vi "ngi request data.vi"(3 "stop":u32, 5 "start":u32, 6 "MAC source":string="\u0000\u0017\r\u0000\u0000`#Ò", 7 "Channels":u8, 8 "error in (no error)":errorcluster, 10 "this instance?":bool=TRUE, 11 "ID":u16) -> (0 "error out":errorcluster)   [LabVIEW 2017]
panel:
  out "concatenated string":string
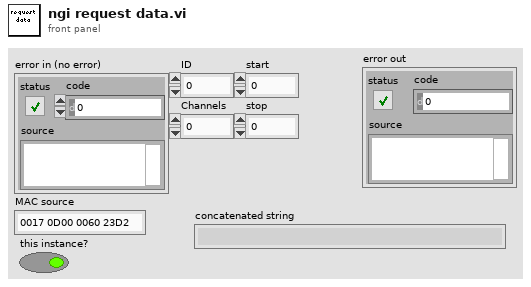
[diagram p1: front panel]
types:
  T1 = cluster{"ID":u16, "Channels":u8, "start":u32, "stop":u32}
  T2 = enum16{"big-endian, network order", "native, host order", "little-endian"}
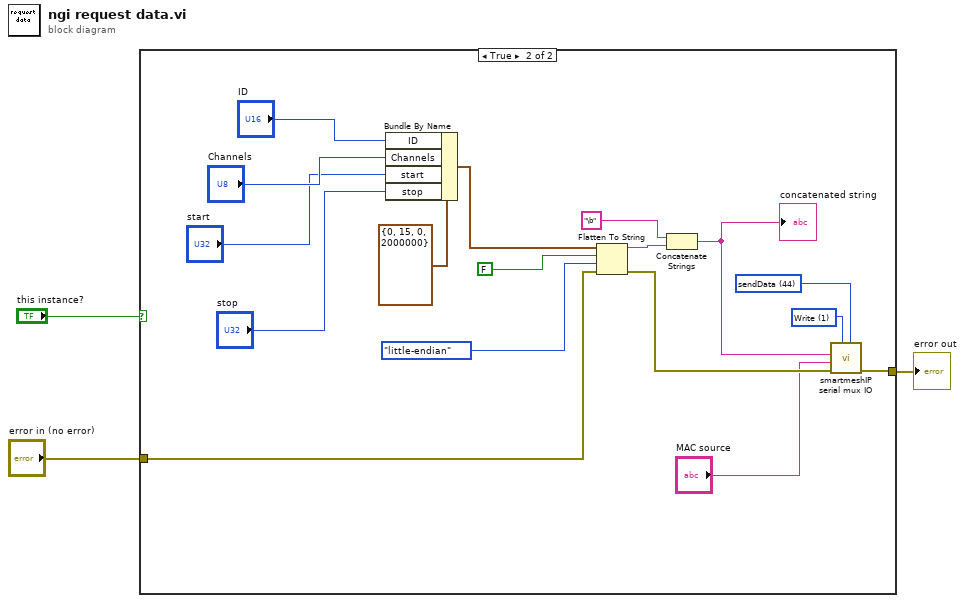
[diagram p0: block diagram]
diagram:
  n1 = case shown="True" "this instance?" {
    tunnel: [w4 w11] -> w3
    tunnel: "error in (no error)" -> [w4 w10]
    frame False {
    }
    frame True {
      w14 = u8 44 items=["subscribe"=22, "startNetwork"=45, "setUser"=58, "setTime"=54, "setNetworkConfig"=26, "setLicense"=56, "setIPConfig"=68, "setDownstreamFrameMode"=51, "setCommonJoinKey"=66, "setAdvertising"=50, "setACLEntry"=39, "sendIP"=59, "sendData"=44, "restorFactoryDefaults"=61, "reset"=21, "radiotestTx"=35, "radiotestRx"=37, "pingMote"=42, "getTime"=23, "getSystemInfo"=46, "radiotestStatistics"=38, "getPathInfo"=48, "getNextPath"=49, "getNextACLEntry"=40, "getNetworkInfo"=64, "getNetworkConfig"=63, "getMoteLinks"=70, "getMoteInfo"=62, "getMoteConfigByld"=65, "getMoteConfig"=47, "getManagerStatistics"=53, "getLog"=43, "getLicense"=55, "getIPConfig"=67, "exchangeNetworkID"=34, "exchangeMoteJoinKey"=33, "deleteMote"=69, "deleteACLEntry"=41, "clearStatistics"=31] ("commandType_write")
      w13 = u16 1 items=["Connect", "Write", "Read", "Close"] ("State")
      n2 = Bundle By Name(cluster=T1 {"ID"=0, "Channels"=15, "start"=0, "stop"=2000000} ("get data 2"), "ID"="ID", "Channels"="Channels", "start"="start", "stop"="stop") -> (w20:T1)
      n3 = Flatten To String(anything=w20, prepend array or string size? (T)=FALSE, byte order (0:big-endian, network order)=T2."little-endian", error in (no error)=w10) -> (data string=w15:string, error out=w12:errorcluster)  [unwired: 1 out]
      n4 = Concatenate Strings("\b", w15) -> (w21:string)
      "concatenated string" <- w21
      n5 = call "smartmeshIP serial mux IO.vi"("tx_commandType"=w14, "State"=w13, "error in"=w12, "MAC source"="MAC source", "tx_data"=w21) -> ("error out"=w11:errorcluster)  [unwired: 1 in, 5 out]
    }
  }
  "error out" <- w3
